vi "LoadingBar.vi"() -> (3 "This VI":refnum<vi>)   [LabVIEW 2014]
panel:
  in  "Loading...":refnum<k7>(container)
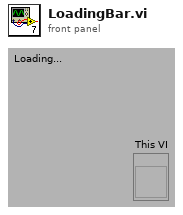
[diagram p1: front panel]
types:
  T1 = enum32{"Invalid", "Standard", "Closed", "Hidden", "Minimized", "Maximized"}
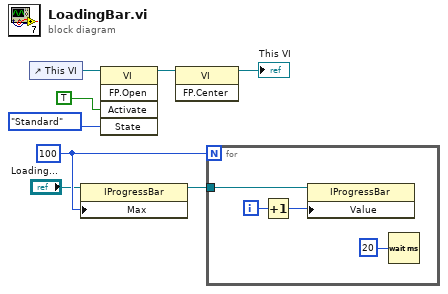
[diagram p0: block diagram]
diagram:
  w8 = 100
  n1 = control-ref of="This VI"() -> (w2:refnum<vi>)
  n2 = property class="IProgressBar"(reference="Loading...", "Max"=w8) -> (reference out=w6:refnum<k7>)  [unwired: 1 in, 1 out]
  n3 = invoke class="VI" method="FP.Open"(reference=w2, "Activate"=TRUE ("Activate?"), "State"=T1."Standard") -> (reference out=w5:refnum<vi>)  [unwired: 2 in, 4 out]
  n4 = invoke class="VI" method="FP.Center"(reference=w5) -> (reference out=→"This VI":refnum<vi>)  [unwired: 2 in, 2 out]
  n5 = for {
    N: w8 -> [_]
    tunnel: w6 -> [w9]
    i -> [w12]
    n6 = Increment(x=w12) -> (x+1=w11:i32)
    n7 = property class="IProgressBar"(reference=w9, "Value"=w11) -> ()  [unwired: 1 in, 2 out]
    n8 = Wait (ms)(milliseconds to wait=u32 20) -> ()  [unwired: 1 out]
  }
